vi "Update_xPos.vi"(7 "NumOfAxis":i32, 8 "error in (no error)":errorcluster, 11 "VISA resource name":refnum<visa-resource-name>) -> (0 "error out":errorcluster, 1 "x_Moving":bool, 2 "Position":dbl[](array[numeric]), 3 "tickcount_pos":u32)   [LabVIEW 2014, in "GRBLMotionCore.lvlib"]
doc: "Performs an instrument error query before terminating the software connection to the instrument."
uses:
  <instrlib>/GRBL/GRBLMotionCore.lvlib
  <instrlib>/GRBL/Public/Position_GRBL.vi
  <vilib>/regexp/Match Regular Expression.xnode
panel:
  out "Read Buffer":string
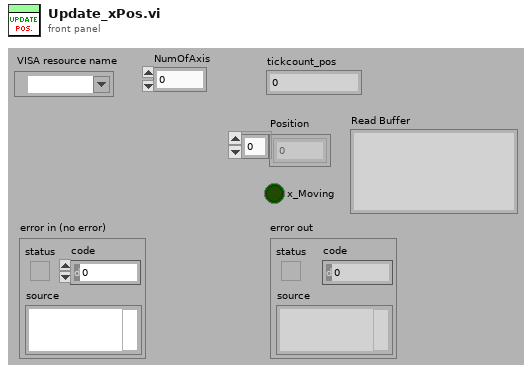
[diagram p1: front panel]
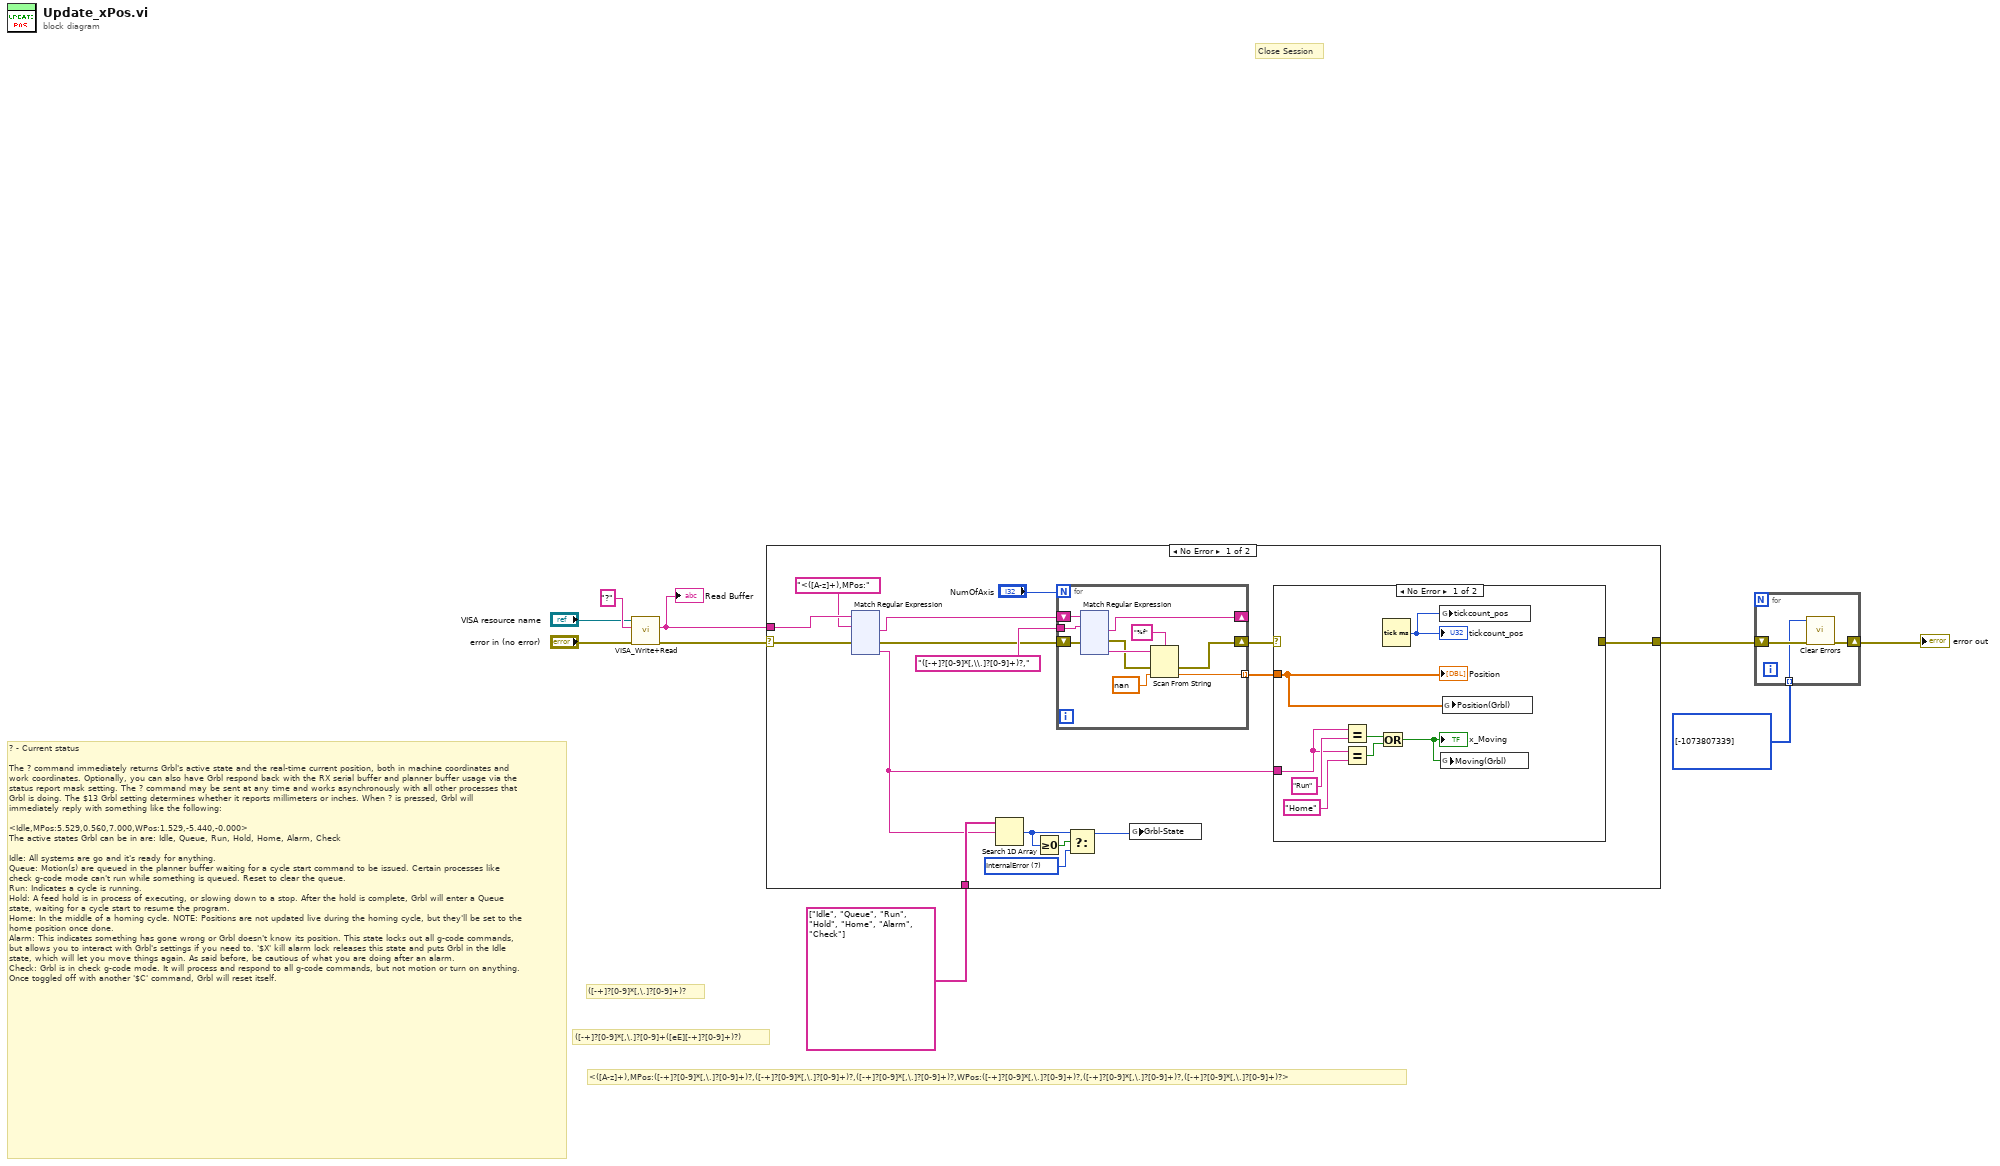
[diagram p0: block diagram]
diagram:
  # "<([A-z]+),MPos:([-+]?[0-9]*[,\\.]?[0-9]+)?,([-+]?[0-9]*[,\\.]?[0-9]+)?,([-+]?[0-9]*[,\\.]?[0-9]+)?,WPos:([-+]?[0-9]*[,\\.]?[0-9]+)?,([-+]?[0-9]*[,\\.]?[0-9]+)?,([-+]?[0-9]*[,\\.]?[0-9]+)?>"
  # "([-+]?[0-9]*[,\\.]?[0-9]+([eE][-+]?[0-9]+)?)"
  # "([-+]?[0-9]*[,\\.]?[0-9]+)?"
  # "? - Current status\n\nThe ? command immediately returns Grbl's active state and the real-time current position, both in machine coordinates and work coordinates. Optionally, you can also have Grbl respond back with the RX serial buffer and planner buffer usage via the status report mask setting. The ? command may be sent at any time and works asynchronously with all other processes that Grbl is doing. The $13 Grbl setting determines whether it reports millimeters or inches. When ? is pressed, Grbl will immediately reply with something like the following:\n\n<Idle,MPos:5.529,0.560,7.000,WPos:1.529,-5.440,-0.000>\nThe active states Grbl can be in are: Idle, Queue, Run, Hold, Home, Alarm, Check\n\nIdle: All systems are go and it's ready for anything.\nQueue: Motion(s) are queued in the planner buffer waiting for a cycle start command to be issued. Certain processes like check g-code mode can't run while something is queued. Reset to clear the queue.\nRun: Indicates a cycle is running.\nHold: A feed hold is in process of executing, or slowing down to a stop. After the hold is complete, Grbl will enter a Queue state, waiting for a cycle start to resume the program.\nHome: In the middle of a homing cycle. NOTE: Positions are not updated live during the homing cycle, but they'll be set to the home position once done.\nAlarm: This indicates something has gone wrong or Grbl doesn't know its position. This state locks out all g-code commands, but allows you to interact with Grbl's settings if you need to. '$X' kill alarm lock releases this state and puts Grbl in the Idle state, which will let you move things again. As said before, be cautious of what you are doing after an alarm.\nCheck: Grbl is in check g-code mode. It will process and respond to all g-code commands, but not motion or turn on anything. Once toggled off with another '$C' command, Grbl will reset itself."
  # "Close Session"
  n1 = call <instrlib>:"VISA_Write+Read.vi"("error in (no error)"="error in (no error)", "Write Buffer"="?" ("string"), "VISA resource name"="VISA resource name") -> ("error out"=w2:errorcluster, "readout"=w8:string)  [unwired: 6 in, 1 out]
  "Read Buffer" <- w8
  n2 = case shown="No Error" w2 {
    selector: w2 -> [w19 w274]
    tunnel: w8 -> [w20 _]
    tunnel: [w21 w274] -> w5
    tunnel: string[] ["Idle", "Queue", "Run", "Hold", "Home", "Alarm", "Check"] ("1D array") -> [w16 _]
    frame No Error {
      w11 = 7 items=["Idle", "Queue", "Run", "Hold", "Home", "Alarm", "Check", "InternalError"] ("Grbl-State")
      n3 = xnode "Match Regular Expression"("input string"=w20, "regular expression"="<([A-z]+),MPos:", "error in"=w19) -> ("after match"=w18:string, "error out"=w10:errorcluster, "submatch 1"=w15:string)  [unwired: 3 in, 3 out]
      n4 = Search 1D Array(1D array=w16, element=w15) -> (index of element=w12:i32)  [unwired: 1 in]
      n5 = Greater Or Equal To 0?(x=w12) -> (x >= 0?=w13:bool)
      n6 = for {
        N: "NumOfAxis" -> [_]
        shift-right: [w159] -> _
        shift-left: w18 -> [w160]
        tunnel: "([-+]?[0-9]*[,\\.]?[0-9]+)?," ("regular expression") -> [w158]
        tunnel: [w156] -> w23 mode=indexing
        shift-right: [w154] -> w22
        shift-left: w10 -> [w152]
        n7 = xnode "Match Regular Expression"("input string"=w160, "regular expression"=w158, "error in"=w152) -> ("after match"=w159:string, "error out"=w153:errorcluster, "submatch 1"=w157:string)  [unwired: 3 in, 3 out]
        n8 = Scan From String(format string="%f", input string=w157, error in=w153, default 1=nan ("default value 1")) -> (error out=w154:errorcluster, output 1=w156:dbl)  [unwired: 1 in, 2 out]
      }
      n9 = Select(t=w12, s=w13, f=w11) -> (s? t:f=w14:i32)
      n10 = global write "Position_GRBL.vi" "Grbl-State"(w14) -> ()
      n11 = case shown="No Error" w22 {
        selector: w22 -> [_ w150]
        tunnel: w23 -> [w148 _]
        tunnel: [_ w150] -> w21
        tunnel: w15 -> [w145 _]
        frame No Error {
          n12 = Equal?(x=w145, y="Run" ("submatch 1")) -> (x = y?=w144:bool)
          n13 = Equal?(x=w145, y="Home" ("submatch 1")) -> (x = y?=w143:bool)
          n14 = Or(x=w144, y=w143) -> (x .or. y?=w142:bool)
          "x_Moving" <- w142
          n15 = Tick Count (ms)() -> (millisecond timer value=w149:u32)
          "tickcount_pos" <- w149
          n16 = global write "Position_GRBL.vi" "tickcount_pos"(w149) -> ()
          n17 = global write "Position_GRBL.vi" "Moving(Grbl)"(w142) -> ()
          n18 = global write "Position_GRBL.vi" "Position(Grbl)"(w148) -> ()
          "Position" <- w148
        }
        frame Error {
          # "removed visa clear ??"
        }
      }
    }
    frame Error {
    }
  }
  n19 = for {
    tunnel: i32[] [-1073807339] -> [w275] mode=indexing
    shift-right: [w277] -> w6
    shift-left: w5 -> [w276]
    n20 = call <vilib>:"Clear Errors.vi"("error in (no error)"=w276, "specific error code to clear (0: all)"=w275) -> ("error out"=w277:errorcluster)  [unwired: 4 in, 1 out]
  }
  "error out" <- w6
